vi "GV DO3.vi"() -> ()   [LabVIEW 2017]
panel:
  out "DO3":bool
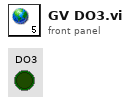
[diagram p1: front panel]
diagram:
